vi "Subtract.vi"(1 "B":dbl, 2 "A":dbl) -> (0 "Sum":dbl)   [LabVIEW 2014]
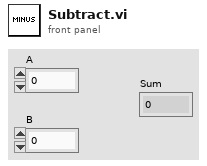
[diagram p1: front panel]
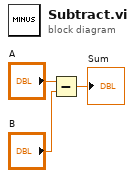
[diagram p0: block diagram]
diagram:
  n1 = Subtract(x="A", y="B") -> (x-y=→"Sum":dbl)
